vi "Set Pin.vi"(0 "Simulated in":refnum<class "Simulated.lvclass">, 5 "VISA resource name":refnum<visa-resource-name>, 7 "Pin":u8, 9 "Pin State":bool, 11 "error in (no error)":errorcluster) -> (4 "Simulated out":refnum<class "Simulated.lvclass">, 6 "VISA resource name 2":refnum<visa-resource-name>, 10 "Command send":string, 15 "error out":errorcluster)   [LabVIEW 2020, in "Simulated.lvclass"]
doc: "Set Pin de un microcontrolador Simulado\nTe da una respuesta simulada en string de lo que estaría recibiendo labview de un microcontrolador fisico"
uses:
  Simulated.lvclass
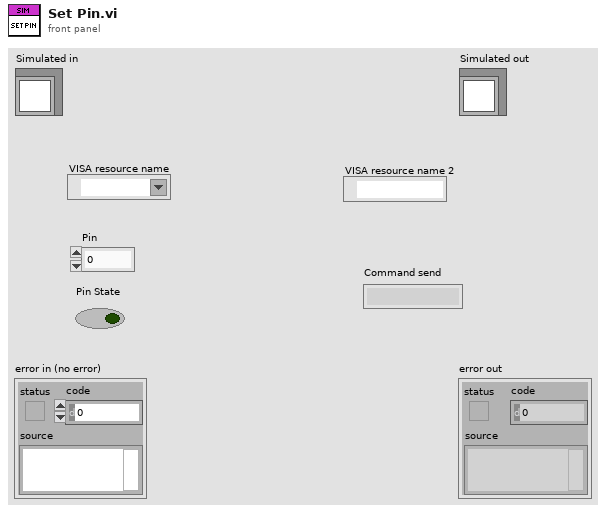
[diagram p1: front panel]
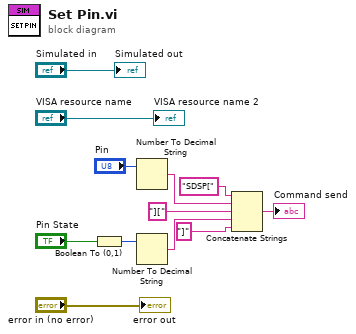
[diagram p0: block diagram]
diagram:
  n1 = Boolean To (0,1)(Boolean="Pin State") -> (0, 1=w4:i16)
  n2 = Number To Decimal String(number="Pin") -> (decimal integer string=w7:string)  [unwired: 1 in]
  n3 = Number To Decimal String(number=w4) -> (decimal integer string=w3:string)  [unwired: 1 in]
  n4 = Concatenate Strings("SDSP[" ("string"), w7, "][" ("string"), w3, "]" ("string")) -> (→"Command send":string)
  "error out" <- "error in (no error)"
  "Simulated out" <- "Simulated in"
  "VISA resource name 2" <- "VISA resource name"
